vi "Get Test Registration by Key.vi"(8 "error in (no error)":errorcluster, 10 "Key":string, 11 "Test Event Storage in":refnum<class "Test Event Storage.lvclass">) -> (0 "error out":errorcluster, 1 "Test Node":T1={"Test Registration"={"Name"="", "Call Chain"=[], "Time Stamp"=timestamp(0 s since 1904-01-01), "Test ID"="", "Caller ID"=""}, "Defined"=TRUE, "Passed"=TRUE}, 2 "Found?":bool, 3 "Test Event Storage out":refnum<class "Test Event Storage.lvclass">)   [LabVIEW 2013, in "Caraya.lvlib" / "Test Event Storage.lvclass"]
uses:
  Test Event Storage.lvclass
  Test Result/Test Node.ctl
  Test Result/Test Registration Data.ctl
  Test Event Storage.lvclass/Test Event Storage.ctl
  Test Result/Test Result.lvclass
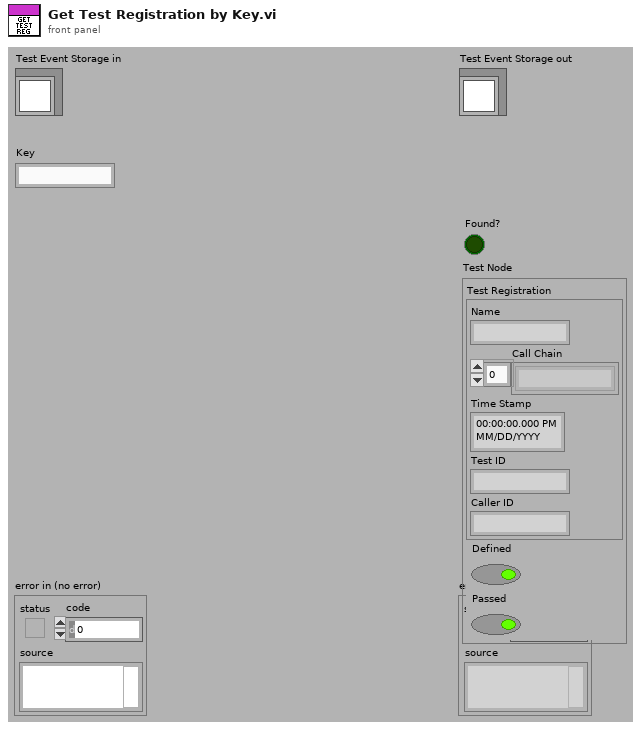
[diagram p1: front panel]
types:
  T1 = typedef "Caraya.lvlib/Test Result.lvclass/Test Node.ctl" = cluster{"Test Registration":T2, "Defined":bool, "Passed":bool}
  T2 = typedef "Caraya.lvlib/Test Result.lvclass/Test Registration Data.ctl" = cluster{"Name":string, "Call Chain":string[], "Time Stamp":timestamp, "Test ID":string, "Caller ID":string}
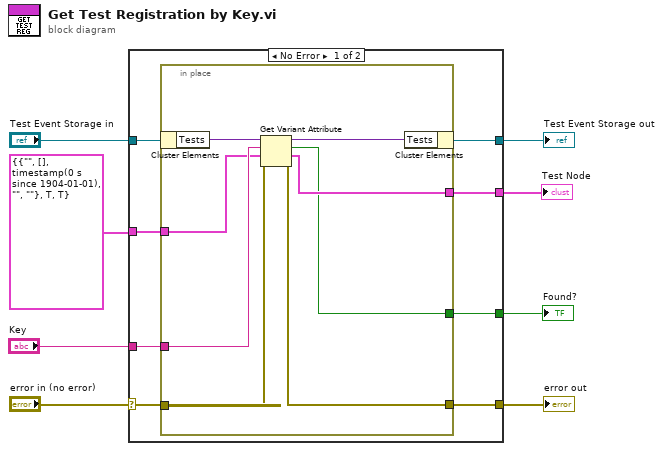
[diagram p0: block diagram]
diagram:
  n1 = case shown="No Error" "error in (no error)" {
    selector: "error in (no error)" -> [w10 w26]
    tunnel: [w16 w26] -> w7
    tunnel: [w15 w25] -> w5
    tunnel: "Test Event Storage in" -> [w12 w25]
    tunnel: T1 {"Test Registration"={"Name"="", "Call Chain"=[], "Time Stamp"=timestamp(0 s since 1904-01-01), "Test ID"="", "Caller ID"=""}, "Defined"=TRUE, "Passed"=TRUE} ("Test Node") -> [w14 _]
    tunnel: [w13 _] -> w1
    tunnel: "Key" -> [w11 _]
    tunnel: [w9 _] -> w3
    frame No Error {
      n2 = in-place {
        in-place-border: w10 -> [w23]
        in-place-border: [w20] -> w16
        in-place-border: w14 -> [w17]
        in-place-border: [w21] -> w13
        in-place-border: w11 -> [w19]
        in-place-border: [w18] -> w9
        n3 = in-place-cluster #1(w12) -> ("Tests"=w24:variant)
        n4 = Get Variant Attribute(Variant=w24, name=w19, default value (empty Variant)=w17, error in=w23) -> (duplicate Variant=w22:variant, found=w18:bool, value=w21:T1, error out=w20:errorcluster)
        n5 = in-place-cluster #1("Tests"=w22) -> (w15:refnum<class "Test Event Storage.lvclass">)
      }
    }
    frame Error {
    }
  }
  "error out" <- w7
  "Test Event Storage out" <- w5
  "Test Node" <- w1
  "Found?" <- w3
